vi "NT_TypeToTypeStr.vi"(11 "type":u32) -> (3 "typeStr":string)   [LabVIEW 2025]
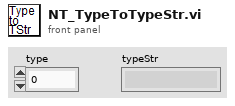
[diagram p1: front panel]
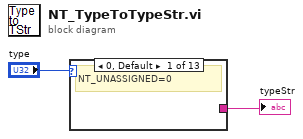
[diagram p0: block diagram]
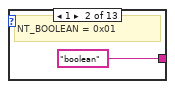
[diagram p2: hidden frame]
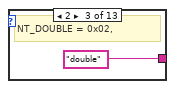
[diagram p3: hidden frame]
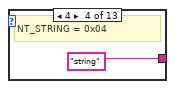
[diagram p4: hidden frame]
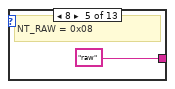
[diagram p5: hidden frame]
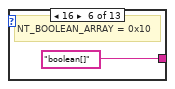
[diagram p6: hidden frame]
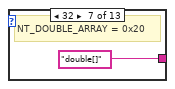
[diagram p7: hidden frame]
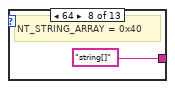
[diagram p8: hidden frame]
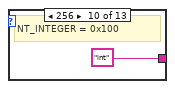
[diagram p10: hidden frame]
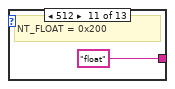
[diagram p11: hidden frame]
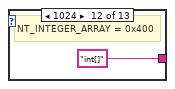
[diagram p12: hidden frame]
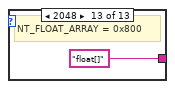
[diagram p13: hidden frame]
diagram:
  n1 = case shown="0, Default" "type" {
    tunnel: [_ "boolean" ("f") "double" ("f") "string" ("f") "raw" ("f") "boolean[]" ("f") "double[]" ("f") "string[]" ("f") _ "int" ("f") "float" ("f") "int[]" ("f") "float[]" ("f")] -> w1
    frame 0, Default {
      # "NT_UNASSIGNED=0"
    }
    frame 1 {
      # "NT_BOOLEAN = 0x01"
    }
    frame 2 {
      # "NT_DOUBLE = 0x02,"
    }
    frame 4 {
      # "NT_STRING = 0x04"
    }
    frame 8 {
      # "NT_RAW = 0x08"
    }
    frame 16 {
      # "NT_BOOLEAN_ARRAY = 0x10"
    }
    frame 32 {
      # "NT_DOUBLE_ARRAY = 0x20"
    }
    frame 64 {
      # "NT_STRING_ARRAY = 0x40"
    }
    frame 128 {
      # "NT_RPC = 0x80"
    }
    frame 256 {
      # "NT_INTEGER = 0x100"
    }
    frame 512 {
      # "NT_FLOAT = 0x200"
    }
    frame 1024 {
      # "NT_INTEGER_ARRAY = 0x400"
    }
    frame 2048 {
      # "NT_FLOAT_ARRAY = 0x800"
    }
  }
  "typeStr" <- w1
